vi "Load New Firmware.vi"(8 "error in":errorcluster) -> (0 "error out":errorcluster, 3 "Return Code":i32)   [LabVIEW 2013]
panel:
  out "appended path":path
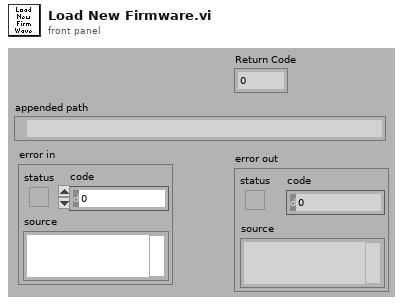
[diagram p1: front panel]
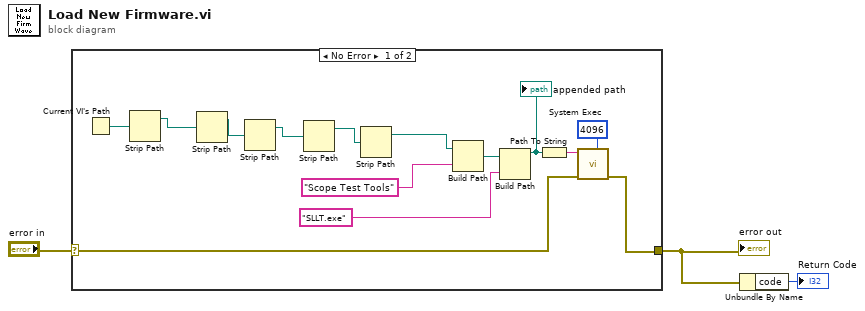
[diagram p0: block diagram]
diagram:
  n1 = case shown="No Error" "error in" {
    selector: "error in" -> [w7 w18]
    tunnel: [w6 w18] -> w2
    frame No Error {
      n2 = Current VI's Path() -> (path=w17:path)
      n3 = Strip Path(path=w17) -> (stripped path=w16:path)  [unwired: 1 out]
      n4 = Strip Path(path=w16) -> (stripped path=w14:path)  [unwired: 1 out]
      n5 = Strip Path(path=w14) -> (stripped path=w15:path)  [unwired: 1 out]
      n6 = Strip Path(path=w15) -> (stripped path=w5:path)  [unwired: 1 out]
      n7 = Strip Path(path=w5) -> (stripped path=w4:path)  [unwired: 1 out]
      n8 = Build Path(base path=w4, name or relative path="Scope Test Tools") -> (appended path=w9:path)
      n9 = Build Path(base path=w9, name or relative path="SLLT.exe") -> (appended path=w10:path)
      "appended path" <- w10
      n10 = Path To String(path=w10) -> (string=w11:string)
      n11 = call <vilib>:"System Exec.vi"("expected output size  (4096)"=u32 4096, "error in (no error)"=w7, "command line"=w11) -> ("error out"=w6:errorcluster)  [unwired: 4 in, 4 out]
    }
    frame Error {
    }
  }
  "error out" <- w2
  n12 = Unbundle By Name(w2) -> ("code"=→"Return Code":i32)
